vi "Wczytaj_wzmA_B_analogowe_INI.vi"(7 "odwroc? (T)":bool=TRUE, 8 "error in (no error)":errorcluster, 11 "Path ini":path=path "C:/Users/user/Documents/Rejestrator/Konfiguracja/dev_27150498.jnj") -> (0 "error out":errorcluster, 1 "HW params":T1={"wsp A"=[[924.40878695, 280.05044565000003, 29.1408959, 3.069102995, 0.31092278139], [914.0777918499999, 281.867210667, 26.882632206700002, 3.0550163421, 0.310968736845], [951.1456429000001, 285.110341112, 27.1990911426, 3.0696112628, 0.31581308595], [914.3476122000001, 281.34234172, 29.109892152, 3.068518068, 0.3126783], [1000.257513479, 304.977147369, 29.713910529099998, 3.0892035357, 0.31184511849999996], [993.0576890607, 303.5092078312, 29.442198783999, 3.0648262983400003, 0.31009064088000005], [1002.5166520152, 305.28578467799997, 29.440497145920002, 3.07102698336, 0.30933858648], [992.737407739, 302.6919371861, 29.47518592865, 3.0793274388799996, 0.31143866215]], "wsp B"=[[924.40878695, 280.05044565000003, 29.1408959, 3.069102995, 0.31092278139], [914.0777918499999, 281.867210667, 26.882632206700002, 3.0550163421, 0.310968736845], [951.1456429000001, 285.110341112, 27.1990911426, 3.0696112628, 0.31581308595], [914.3476122000001, 281.34234172, 29.109892152, 3.068518068, 0.3126783], [1000.257513479, 304.977147369, 29.713910529099998, 3.0892035357, 0.31184511849999996], [993.0576890607, 303.5092078312, 29.442198783999, 3.0648262983400003, 0.31009064088000005], [1002.5166520152, 305.28578467799997, 29.440497145920002, 3.07102698336, 0.30933858648], [992.737407739, 302.6919371861, 29.47518592865, 3.0793274388799996, 0.31143866215]]}, 2 "Wzmocnienia":dbl[][](array[numeric]), 5 "Info":string[](array[string]))   [LabVIEW 2014]
uses:
  Kontrolki/KartaDAQ/A_B konfig params.ctl
  <vilib>/Utility/config.llb/NI_LVConfig.lvlib
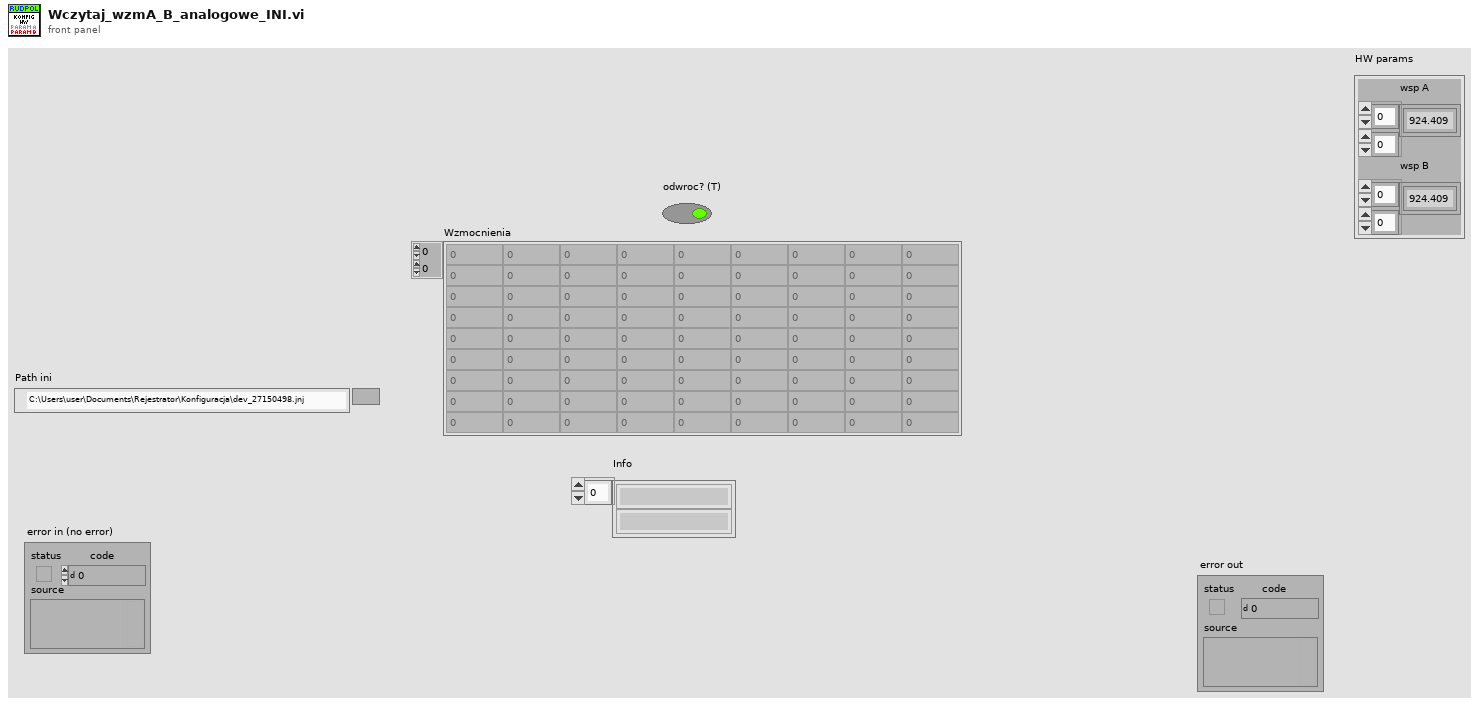
[diagram p1: front panel]
types:
  T1 = typedef "A_B konfig params.ctl" = cluster{"wsp A":dbl[][], "wsp B":dbl[][]}
  T2 = typedef "NI_LVConfig.lvlib/Config Data RefNum.ctl" = refnum<k1>
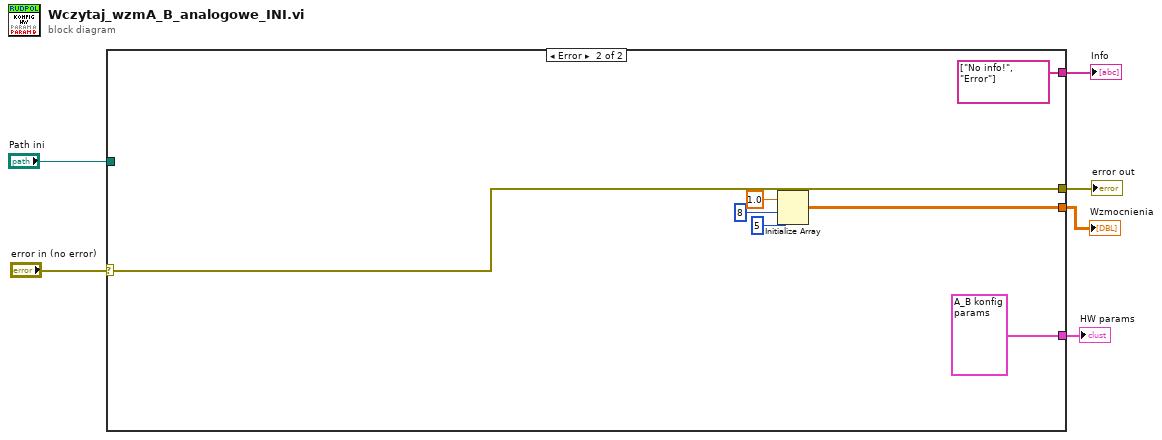
[diagram p0: block diagram]
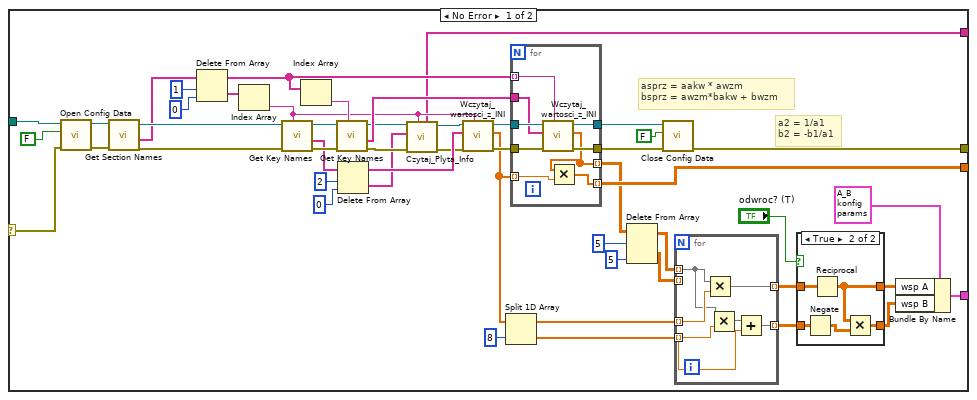
[diagram p2: hidden frame]
diagram:
  n1 = case shown="Error" "error in (no error)" {
    selector: "error in (no error)" -> [w55 w85]
    tunnel: [w49 w85] -> w5
    tunnel: "Path ini" -> [w56 _]
    tunnel: [w30 w81] -> w3
    tunnel: [w15 T1 {"wsp A"=[[924.40878695, 280.05044565000003, 29.1408959, 3.069102995, 0.31092278139], [914.0777918499999, 281.867210667, 26.882632206700002, 3.0550163421, 0.310968736845], [951.1456429000001, 285.110341112, 27.1990911426, 3.0696112628, 0.31581308595], [914.3476122000001, 281.34234172, 29.109892152, 3.068518068, 0.3126783], [1000.257513479, 304.977147369, 29.713910529099998, 3.0892035357, 0.31184511849999996], [993.0576890607, 303.5092078312, 29.442198783999, 3.0648262983400003, 0.31009064088000005], [1002.5166520152, 305.28578467799997, 29.440497145920002, 3.07102698336, 0.30933858648], [992.737407739, 302.6919371861, 29.47518592865, 3.0793274388799996, 0.31143866215]], "wsp B"=[[924.40878695, 280.05044565000003, 29.1408959, 3.069102995, 0.31092278139], [914.0777918499999, 281.867210667, 26.882632206700002, 3.0550163421, 0.310968736845], [951.1456429000001, 285.110341112, 27.1990911426, 3.0696112628, 0.31581308595], [914.3476122000001, 281.34234172, 29.109892152, 3.068518068, 0.3126783], [1000.257513479, 304.977147369, 29.713910529099998, 3.0892035357, 0.31184511849999996], [993.0576890607, 303.5092078312, 29.442198783999, 3.0648262983400003, 0.31009064088000005], [1002.5166520152, 305.28578467799997, 29.440497145920002, 3.07102698336, 0.30933858648], [992.737407739, 302.6919371861, 29.47518592865, 3.0793274388799996, 0.31143866215]]}] -> w2
    tunnel: [w7 string[] ["No info!", "Error"] ("Konfig Info")] -> w1
    frame No Error {
      # "a2 = 1/a1\nb2 = -b1/a1"
      # "asprz = aakw * awzm\nbsprz = awzm*bakw + bwzm"
      n2 = call <vilib>:"Open Config Data.vi"("error in (no error)"=w55, "create file if necessary (T)"=FALSE, "configuration file path"=w56) -> ("error out"=w52:errorcluster, "refnum"=w53:T2)  [unwired: 6 in, 1 out]
      n3 = call <vilib>:"Get Section Names.vi"("error in (no error)"=w52, "refnum"=w53) -> ("error out"=w50:errorcluster, "section names"=w45:string[], "refnum out"=w51:T2)  [unwired: 7 in]
      n4 = Delete From Array ("section names")(array=w45, length=1, index=0) -> (deleted portion=w44:string[], array with subset deleted=w36:string[])
      n5 = Index Array(array=w44) -> (element=w8:string)  [unwired: 1 in]
      n6 = call <vilib>:"Get Key Names.vi"("section"=w8, "error in (no error)"=w50, "refnum"=w51) -> ("error out"=w39:errorcluster, "key names"=w33:string[], "refnum out"=w38:T2)  [unwired: 5 in, 1 out]
      n7 = Index Array(array=w36) -> (element=w37:string)  [unwired: 1 in]
      n8 = call <vilib>:"Get Key Names.vi"("section"=w37, "error in (no error)"=w39, "refnum"=w38) -> ("error out"=w13:errorcluster, "key names"=w32:string[], "refnum out"=w10:T2)  [unwired: 5 in, 1 out]
      n9 = Delete From Array(array=w33, length=2, index=0) -> (deleted portion=w11:string[], array with subset deleted=w14:string[])
      n10 = call "Czytaj_Plyta_Info.vi"("Section"=w8, "error in (no error)"=w13, "key names"=w11, "Refnum in"=w10) -> ("error out"=w12:errorcluster, "Refnum out"=w9:T2, "Konfig Info"=w7:string[])  [unwired: 4 in]
      n11 = call "Wczytaj_wartosci_z_INI.vi"("Section"=w8, "error in (no error)"=w12, "key names"=w14, "refnum"=w9) -> ("error out"=w43:errorcluster, "Array"=w23:dbl[], "refnum out"=w42:T2)  [unwired: 5 in]
      n12 = Split 1D Array(array=w23, index=8) -> (first subarray=w25:dbl[], second subarray=w24:dbl[])
      n13 = for {
        tunnel: w43 -> [w78]
        tunnel: w42 -> [w77]
        tunnel: [w75] -> w41
        tunnel: w36 -> [w74] mode=indexing
        tunnel: w32 -> [w73]
        tunnel: [w76] -> w40
        tunnel: [w72] -> w30 mode=indexing
        tunnel: w23 -> [w71] mode=indexing
        tunnel: [w70] -> w22 mode=indexing
        n14 = call "Wczytaj_wartosci_z_INI.vi"("Section"=w74, "error in (no error)"=w78, "key names"=w73, "refnum"=w77) -> ("error out"=w76:errorcluster, "Array"=w70:dbl[], "refnum out"=w75:T2)  [unwired: 5 in]
        n15 = Multiply(x=w70, y=w71) -> (x*y=w72:dbl[])
      }
      n16 = Delete From Array(array=w22, length=5, index (col)=5 ("disabled index (col)")) -> (deleted portion=w26:dbl[][], array with subset deleted=w27:dbl[][])  [unwired: 1 in]
      n17 = call <vilib>:"Close Config Data.vi"("error in (no error)"=w40, "write file if changed (T)"=FALSE, "refnum"=w41) -> ("error out"=w49:errorcluster)  [unwired: 7 in, 1 out]
      n18 = for {
        tunnel: w27 -> [w67] mode=indexing
        tunnel: w26 -> [_] mode=indexing
        tunnel: w25 -> [w69] mode=indexing
        tunnel: w24 -> [w65] mode=indexing
        tunnel: [w68] -> w21 mode=indexing
        tunnel: [w64] -> w20 mode=indexing
        n19 = Multiply(x=w67, y=w69) -> (x*y=w68:dbl[])
        n20 = Multiply(x=w67, y=w65) -> (x*y=w66:dbl[])
        n21 = Add(x=w66, y=w65) -> (x+y=w64:dbl[])
      }
      n22 = case shown="True" "odwroc? (T)" {
        tunnel: w21 -> [w58 w63]
        tunnel: [w58 w59] -> w17
        tunnel: w20 -> [w57 w62]
        tunnel: [w57 w61] -> w16
        frame False {
        }
        frame True {
          n23 = Negate(x=w62) -> (-x=w60:dbl[][])
          n24 = Reciprocal(x=w63) -> (1/x=w59:dbl[][])
          n25 = Multiply(x=w59, y=w60) -> (x*y=w61:dbl[][])
        }
      }
      n26 = Bundle By Name(cluster=T1 {"wsp A"=[[924.40878695, 280.05044565000003, 29.1408959, 3.069102995, 0.31092278139], [914.0777918499999, 281.867210667, 26.882632206700002, 3.0550163421, 0.310968736845], [951.1456429000001, 285.110341112, 27.1990911426, 3.0696112628, 0.31581308595], [914.3476122000001, 281.34234172, 29.109892152, 3.068518068, 0.3126783], [1000.257513479, 304.977147369, 29.713910529099998, 3.0892035357, 0.31184511849999996], [993.0576890607, 303.5092078312, 29.442198783999, 3.0648262983400003, 0.31009064088000005], [1002.5166520152, 305.28578467799997, 29.440497145920002, 3.07102698336, 0.30933858648], [992.737407739, 302.6919371861, 29.47518592865, 3.0793274388799996, 0.31143866215]], "wsp B"=[[924.40878695, 280.05044565000003, 29.1408959, 3.069102995, 0.31092278139], [914.0777918499999, 281.867210667, 26.882632206700002, 3.0550163421, 0.310968736845], [951.1456429000001, 285.110341112, 27.1990911426, 3.0696112628, 0.31581308595], [914.3476122000001, 281.34234172, 29.109892152, 3.068518068, 0.3126783], [1000.257513479, 304.977147369, 29.713910529099998, 3.0892035357, 0.31184511849999996], [993.0576890607, 303.5092078312, 29.442198783999, 3.0648262983400003, 0.31009064088000005], [1002.5166520152, 305.28578467799997, 29.440497145920002, 3.07102698336, 0.30933858648], [992.737407739, 302.6919371861, 29.47518592865, 3.0793274388799996, 0.31143866215]]}, "wsp A"=w17, "wsp B"=w16) -> (w15:T1)
    }
    frame Error {
      n27 = Initialize Array(1.0 ("element"), 8 ("dimension size"), 5 ("dimension size")) -> (w81:dbl[][])
    }
  }
  "error out" <- w5
  "Wzmocnienia" <- w3
  "HW params" <- w2
  "Info" <- w1
